vi "set control size.vi"(8 "error in (no error)":errorcluster, 10 "Size":T1, 11 "Path Control.lvclass":refnum<class "Path Control.lvclass">) -> (0 "error out":errorcluster, 3 "Path Control.lvclass":refnum<class "Path Control.lvclass">)   [LabVIEW 2010, in "Path Control.lvclass"]
uses:
  Path Control.lvclass
  <vilib>/Utility/miscctls.llb/LVBoundsTypeDef.ctl
  Control/Control.lvclass
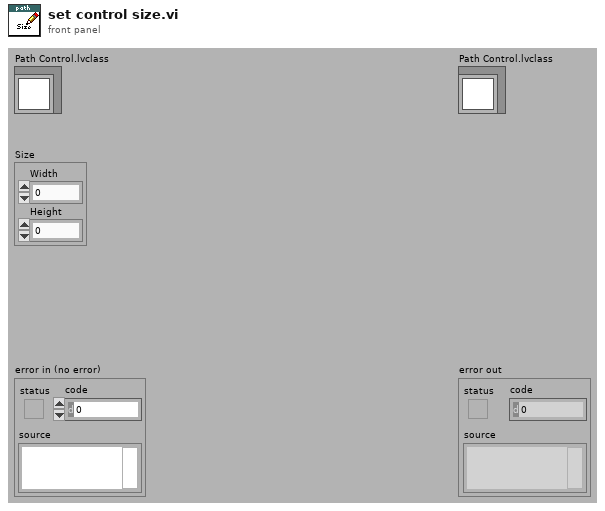
[diagram p1: front panel]
types:
  T1 = typedef "LVBoundsTypeDef.ctl" = cluster{"Width":u32, "Height":u32}
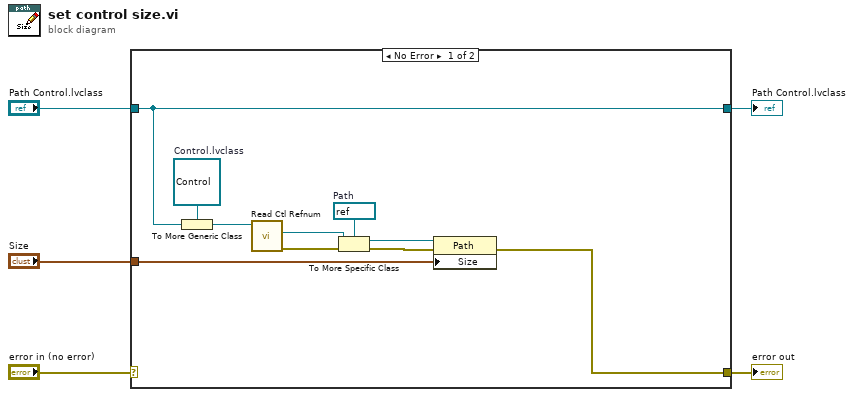
[diagram p0: block diagram]
diagram:
  n1 = case shown="No Error" "error in (no error)" {
    selector: "error in (no error)" -> [_ w17]
    tunnel: [w11 w17] -> w4
    tunnel: [w8 w16] -> w2
    tunnel: "Path Control.lvclass" -> [w8 w16]
    tunnel: "Size" -> [w12 _]
    frame No Error {
      w10 = refnum<class "Control.lvclass"> refnum  # Control.lvclass
      w15 = refnum<vi> refnum  # Path
      n2 = To More Generic Class(target class=w10, reference=w8) -> (generic class reference=w9:refnum<class "Control.lvclass">)
      n3 = call-dynamic "Read Ctl Refnum.vi"("Control in"=w9) -> ("error out"=w6:errorcluster, "Ctl Refnum"=w7:refnum<vi>)  [unwired: 8 in, 1 out]
      n4 = To More Specific Class(target class=w15, reference=w7, error in=w6) -> (specific class reference=w14:refnum<vi>, error out=w13:errorcluster)
      n5 = property class="Path"(reference=w14, error in=w13, "Size"=w12) -> (error out=w11:errorcluster)  [unwired: 1 out]
    }
    frame Error {
    }
  }
  "error out" <- w4
  "Path Control.lvclass" <- w2
